vi "FPGA Write Array - I64.vi"(8 "error in (no error)":errorcluster, 9 "Array":i64[](array[numeric]), 10 "Control":T1, 11 "FPGA Session In":refnum<class "Firmware Independent PID Interface.lvclass">) -> (0 "error out":errorcluster, 3 "FPGA Session Out":refnum<class "Firmware Independent PID Interface.lvclass">)   [LabVIEW 2010, in "Firmware Independent PID Interface.lvclass"]
doc: "Writes an entire array of signed 64-bit integer values to a given array control or indicator."
uses:
  Firmware Independent PID Interface.lvclass
  TypeDefs/ControlArrayI64.ctl
  <vilib>/rvi/DataTransferAndStorage/Container/Common/niFpgaDataTypeControl.ctl
  <userlib>/_FPGA Interface Advanced Tools/FPGA Interface Base/FPGA Interface Base.lvclass/FPGA Interface Base.ctl
  <userlib>/_FPGA Interface Advanced Tools/FPGA Interface Base/Accessors/FPGA Read Session.vi
  <userlib>/_FPGA Interface Advanced Tools/FPGA Interface Wrapper/FPGA Interface Wrapper.lvlib
  <userlib>/_FPGA Interface Advanced Tools/FPGA Interface Base/FPGA Interface Base.lvclass
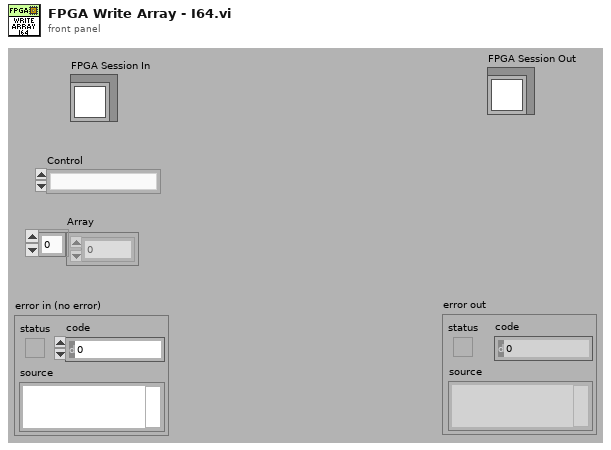
[diagram p1: front panel]
types:
  T1 = typedef "Firmware Independent PID Interface.lvclass/ControlArrayI64.ctl" = enum16{""}
  T2 = typedef "niFpgaDataTypeControl.ctl" = enum32{"Boolean", "I8", "I16", "I32", "I64", "U8", "U16", "U32", "U64", "FXP", "CustomControl"}
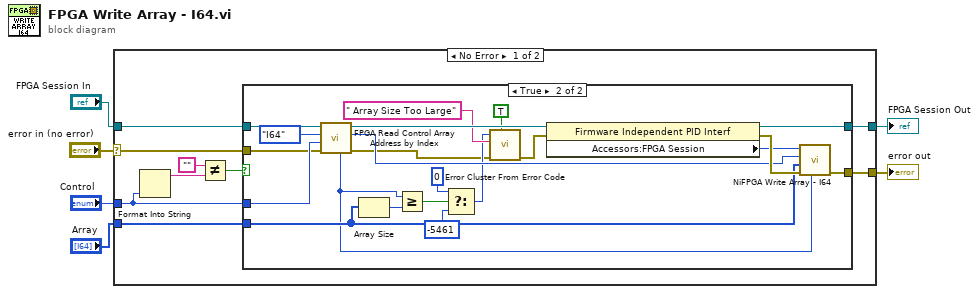
[diagram p0: block diagram]
diagram:
  n1 = case shown="No Error" "error in (no error)" {
    selector: "error in (no error)" -> [w8 w40]
    tunnel: [w10 w40] -> w1
    tunnel: [w9 w39] -> w2
    tunnel: "FPGA Session In" -> [w13 w39]
    tunnel: "Control" -> [w11 _]
    tunnel: "Array" -> [w7 _]
    frame No Error {
      n2 = Format Into String(w11) -> (resulting string=w15:string)  [unwired: 3 in, 1 out]
      n3 = Not Equal?(x="", y=w15) -> (x != y?=w12:bool)
      n4 = case shown="True" w12 {
        tunnel: [w16 w31] -> w10
        tunnel: [w17 w35] -> w9
        tunnel: w13 -> [w17 w36]
        tunnel: w11 -> [_ w34]
        tunnel: w8 -> [w16 w33]
        tunnel: w7 -> [_ w27]
        frame False {
        }
        frame True {
          n5 = call <userlib>:"FPGA Read Control Array Address by Index.vi"("error in (no error)"=w33, "index"=w34, "Data Type"=niFpgaDataTypeControl."I64", "FPGA Interface Base in"=w36) -> ("error out"=w19:errorcluster, "Address"=w29:u32, "FPGA Interface Base out"=w37:refnum<class "Firmware Independent PID Interface.lvclass">, "Num Elements"=w26:u32)  [unwired: 3 in, 1 out]
          n6 = Array Size(array=w27) -> (size(s)=w32:i32)
          n7 = Greater Or Equal?(x=w26, y=w32) -> (x >= y?=w20:bool)
          n8 = Select(t=0, s=w20, f=-5461 ("error code (0)")) -> (s? t:f=w21:i32)
          n9 = call <vilib>:"Error Cluster From Error Code.vi"("show call chain? (False)"=TRUE, "error in (no error)"=w19, "error message (\"\")"=" Array Size Too Large" ("string"), "error code (0)"=w21) -> ("error out"=w18:errorcluster)  [unwired: 5 in]
          n10 = property class="Firmware Independent PID Interf"(reference=w37, error in=w18) -> (reference out=w35:refnum<class "Firmware Independent PID Interface.lvclass">, error out=w30:errorcluster, "Accessors:FPGA Session"=w28:u32)
          n11 = call <userlib>:"NiFPGA Write Array - I64.vi"("Size"=w26, "error in (no error)"=w30, "Array"=w27, "Control"=w29, "Session"=w28) -> ("error out"=w31:errorcluster)  [unwired: 5 in, 1 out]
        }
      }
    }
    frame Error {
    }
  }
  "error out" <- w1
  "FPGA Session Out" <- w2
